vi "SSC DCPower Configure Output Enabled And Connected V3.vi"(0 "DCPower SSC in":T1[](array[typedef]), 5 "Output Enabled And Connected":bool, 7 "Delay Before/After VDD":dbl format="%#_6p", 11 "error in":errorcluster) -> (4 "DCPower SSC out":T1[](array[typedef]), 15 "error out":errorcluster)   [LabVIEW 2019]
doc: "This VI configures output enabled and connected on the channels.\n\nT - Enable and then connect\nF - Disconnect and then disable"
uses:
  SSC DCPower.ctl
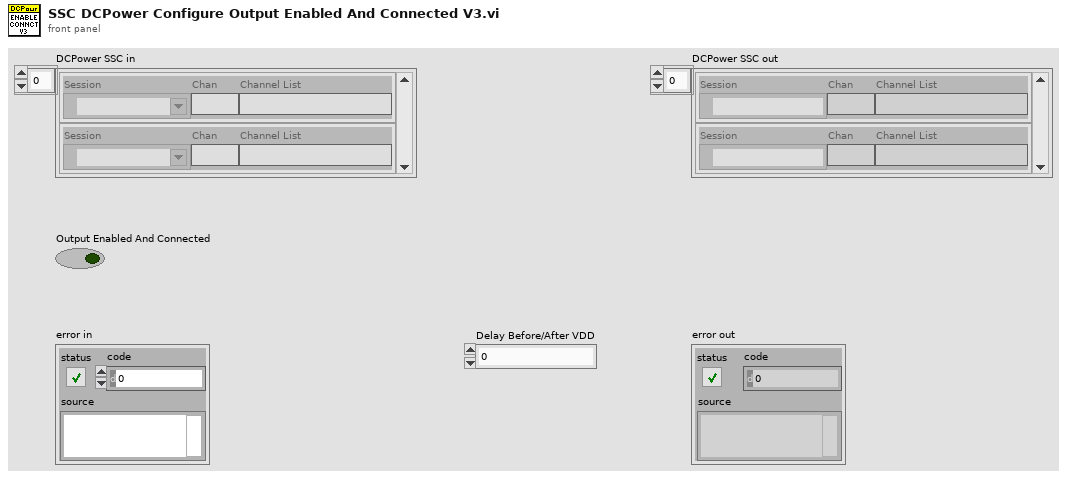
[diagram p1: front panel]
types:
  T1 = typedef "SSC DCPower.ctl" = cluster{"Session":refnum<k15>, "Chan":string, "Channel List":string}
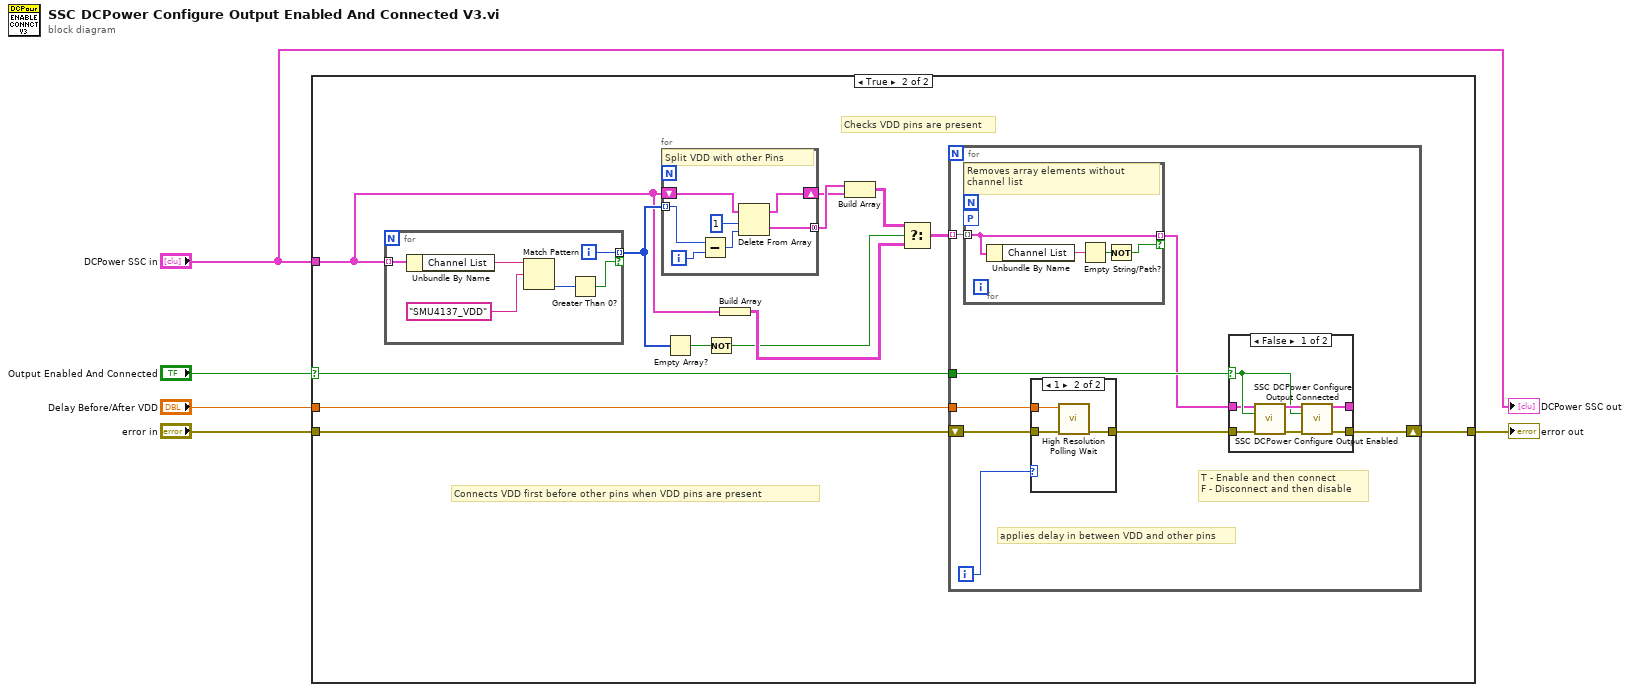
[diagram p0: block diagram]
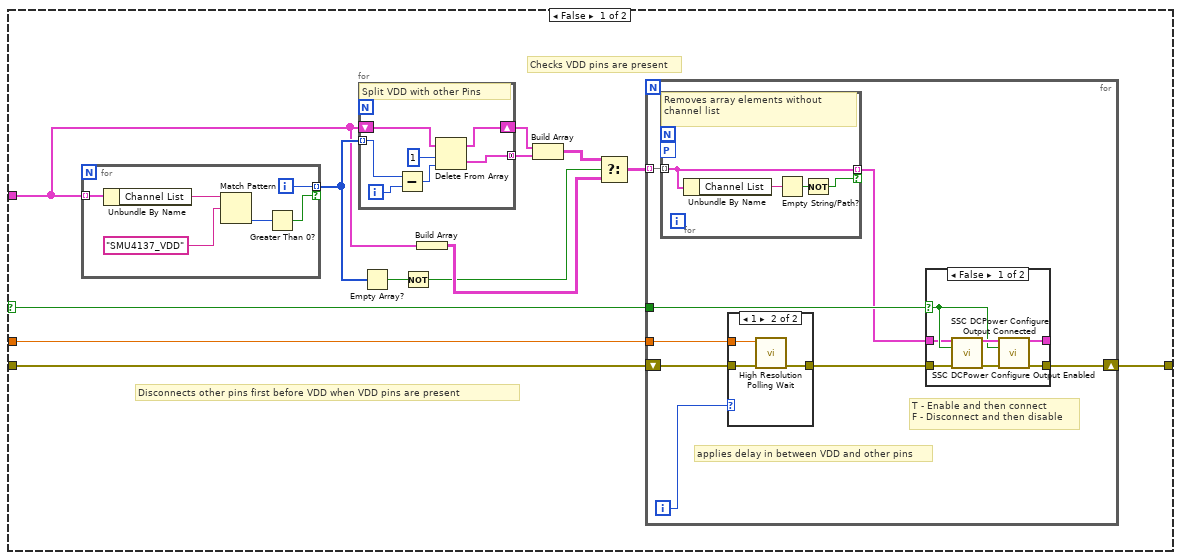
[diagram p2: hidden frame]
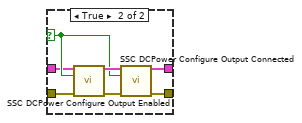
[diagram p4: hidden frame]
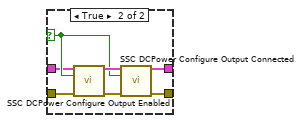
[diagram p6: hidden frame]
diagram:
  n1 = case shown="True" "Output Enabled And Connected" {
    selector: "Output Enabled And Connected" -> [w7 w65]
    tunnel: "error in" -> [w12 w68]
    tunnel: [w10 w66] -> w4
    tunnel: "DCPower SSC in" -> [w11 w67]
    tunnel: "Delay Before/After VDD" -> [w6 w64]
    frame False {
      # "Disconnects other pins first before VDD when VDD pins are present"
      # "Checks VDD pins are present"
      n2 = for {
        tunnel: w11 -> [w31] mode=indexing
        tunnel: [w27] -> w18 mode=indexing if=w26
        i -> [w27]
        n3 = Unbundle By Name(w31) -> ("Channel List"=w30:string)
        n4 = Match Pattern(string=w30, regular expression="SMU4137_VDD") -> (offset past match=w28:i32)  [unwired: 1 in, 3 out]
        n5 = Greater Than 0?(x=w28) -> (x > 0?=w26:bool)
      }
      n6 = for {
        shift-right: [w22] -> w9
        shift-left: w11 -> [w25]
        tunnel: w18 -> [w21] mode=indexing
        tunnel: [w24] -> w8 mode=concatenating
        i -> [w19]
        # "Split VDD with other Pins"
        n7 = Subtract(x=w21, y=w19) -> (x-y=w20:i32)
        n8 = Delete From Array(array=w25, length=1, index=w20) -> (deleted portion=w24:T1[], array with subset deleted=w22:T1[])
      }
      n9 = Empty Array?(array=w18) -> (empty?=w17:bool)
      n10 = Not(x=w17) -> (.not. x?=w14:bool)
      n11 = Build Array(w11) -> (w15:T1[][])
      n12 = Build Array(w9, w8) -> (w16:T1[][])
      n13 = Select(t=w16, s=w14, f=w15) -> (s? t:f=w13:T1[][])
      n14 = for {
        tunnel: w7 -> [w39]
        shift-right: [w32] -> w10
        shift-left: w12 -> [w37]
        tunnel: w13 -> [w38] mode=indexing
        tunnel: w6 -> [w36]
        i -> [w35]
        # "applies delay in between VDD and other pins"
        # "T - Enable and then connect\nF - Disconnect and then disable"
        n15 = for {
          tunnel: w38 -> [w47] mode=indexing
          workers-P: _ -> [_]
          tunnel: [w47] -> w33 mode=indexing if=w44
          # "Removes array elements without channel list"
          n16 = Unbundle By Name(w47) -> ("Channel List"=w45:string)
          n17 = Empty String/Path?(string/path=w45) -> (empty?=w46:bool)
          n18 = Not(x=w46) -> (.not. x?=w44:bool)
        }
        n19 = case shown="1" w35 {
          tunnel: w37 -> [w40 w43]
          tunnel: [w40 w42] -> w34
          tunnel: w36 -> [_ w41]
          frame 0, Default {
          }
          frame 1 {
            n20 = call <vilib>:"High Resolution Polling Wait.vi"("error in (no error)"=w43, "seconds to wait"=w41) -> ("error out"=w42:errorcluster)  [unwired: 9 in]
          }
        }
        n21 = case shown="False" w39 {
          selector: w39 -> [w49 w56]
          tunnel: w34 -> [w54 w61]
          tunnel: [w52 w59] -> w32
          tunnel: [w50 w57] -> _
          tunnel: w33 -> [w48 w55]
          frame False {
            n22 = call "SSC DCPower Configure Output Connected.vi"("DCPower SSC in"=w48, "Output Connected"=w49, "error in"=w54) -> ("DCPower SSC out"=w51:T1[], "error out"=w53:errorcluster)  [unwired: 11 in]
            n23 = call "SSC DCPower Configure Output Enabled.vi"("DCPower SSC in"=w51, "Output Enabled"=w49, "error in"=w53) -> ("DCPower SSC out"=w50:T1[], "error out"=w52:errorcluster)  [unwired: 11 in]
          }
          frame True {
            n24 = call "SSC DCPower Configure Output Enabled.vi"("DCPower SSC in"=w55, "Output Enabled"=w56, "error in"=w61) -> ("DCPower SSC out"=w58:T1[], "error out"=w60:errorcluster)  [unwired: 11 in]
            n25 = call "SSC DCPower Configure Output Connected.vi"("DCPower SSC in"=w58, "Output Connected"=w56, "error in"=w60) -> ("DCPower SSC out"=w57:T1[], "error out"=w59:errorcluster)  [unwired: 11 in]
          }
        }
      }
    }
    frame True {
      # "Connects VDD first before other pins when VDD pins are present"
      # "Checks VDD pins are present"
      n26 = for {
        tunnel: w67 -> [w87] mode=indexing
        tunnel: [w83] -> w74 mode=indexing if=w82
        i -> [w83]
        n27 = Unbundle By Name(w87) -> ("Channel List"=w86:string)
        n28 = Match Pattern(string=w86, regular expression="SMU4137_VDD") -> (offset past match=w84:i32)  [unwired: 1 in, 3 out]
        n29 = Greater Than 0?(x=w84) -> (x > 0?=w82:bool)
      }
      n30 = for {
        shift-right: [w78] -> w62
        shift-left: w67 -> [w81]
        tunnel: w74 -> [w77] mode=indexing
        tunnel: [w80] -> w63 mode=concatenating
        i -> [w75]
        # "Split VDD with other Pins"
        n31 = Subtract(x=w77, y=w75) -> (x-y=w76:i32)
        n32 = Delete From Array(array=w81, length=1, index=w76) -> (deleted portion=w80:T1[], array with subset deleted=w78:T1[])
      }
      n33 = Empty Array?(array=w74) -> (empty?=w73:bool)
      n34 = Not(x=w73) -> (.not. x?=w70:bool)
      n35 = Build Array(w67) -> (w71:T1[][])
      n36 = Build Array(w63, w62) -> (w72:T1[][])
      n37 = Select(t=w72, s=w70, f=w71) -> (s? t:f=w69:T1[][])
      n38 = for {
        tunnel: w65 -> [w95]
        shift-right: [w88] -> w66
        shift-left: w68 -> [w93]
        tunnel: w69 -> [w94] mode=indexing
        tunnel: w64 -> [w92]
        i -> [w91]
        # "applies delay in between VDD and other pins"
        # "T - Enable and then connect\nF - Disconnect and then disable"
        n39 = for {
          tunnel: w94 -> [w103] mode=indexing
          workers-P: _ -> [_]
          tunnel: [w103] -> w89 mode=indexing if=w100
          # "Removes array elements without channel list"
          n40 = Unbundle By Name(w103) -> ("Channel List"=w101:string)
          n41 = Empty String/Path?(string/path=w101) -> (empty?=w102:bool)
          n42 = Not(x=w102) -> (.not. x?=w100:bool)
        }
        n43 = case shown="1" w91 {
          tunnel: w93 -> [w96 w99]
          tunnel: [w96 w98] -> w90
          tunnel: w92 -> [_ w97]
          frame 0, Default {
          }
          frame 1 {
            n44 = call <vilib>:"High Resolution Polling Wait.vi"("error in (no error)"=w99, "seconds to wait"=w97) -> ("error out"=w98:errorcluster)  [unwired: 9 in]
          }
        }
        n45 = case shown="False" w95 {
          selector: w95 -> [w105 w112]
          tunnel: w90 -> [w110 w117]
          tunnel: [w108 w115] -> w88
          tunnel: [w106 w113] -> _
          tunnel: w89 -> [w104 w111]
          frame False {
            n46 = call "SSC DCPower Configure Output Connected.vi"("DCPower SSC in"=w104, "Output Connected"=w105, "error in"=w110) -> ("DCPower SSC out"=w107:T1[], "error out"=w109:errorcluster)  [unwired: 11 in]
            n47 = call "SSC DCPower Configure Output Enabled.vi"("DCPower SSC in"=w107, "Output Enabled"=w105, "error in"=w109) -> ("DCPower SSC out"=w106:T1[], "error out"=w108:errorcluster)  [unwired: 11 in]
          }
          frame True {
            n48 = call "SSC DCPower Configure Output Enabled.vi"("DCPower SSC in"=w111, "Output Enabled"=w112, "error in"=w117) -> ("DCPower SSC out"=w114:T1[], "error out"=w116:errorcluster)  [unwired: 11 in]
            n49 = call "SSC DCPower Configure Output Connected.vi"("DCPower SSC in"=w114, "Output Connected"=w112, "error in"=w116) -> ("DCPower SSC out"=w113:T1[], "error out"=w115:errorcluster)  [unwired: 11 in]
          }
        }
      }
    }
  }
  "error out" <- w4
  "DCPower SSC out" <- "DCPower SSC in"
